vi "ReadWrite.ProcessData.vi"(8 "error in (no error)":errorcluster, 10 "timeout ms":i32=100, 11 "ReadWrite in":refnum<class "ReadWrite.lvclass">) -> (0 "error out":errorcluster, 1 "Timeout?":bool, 2 "Values":dbl[](array[numeric]), 3 "ReadWrite out":refnum<class "ReadWrite.lvclass">, 5 "Detect?":bool[](array[boolean]))   [LabVIEW 2023, in "Plugin Data Access Engine.lvlib" / "ReadWrite.lvclass"]
uses:
  ReadWrite.lvclass
  ReadWrite.lvclass/ReadWrite.ctl
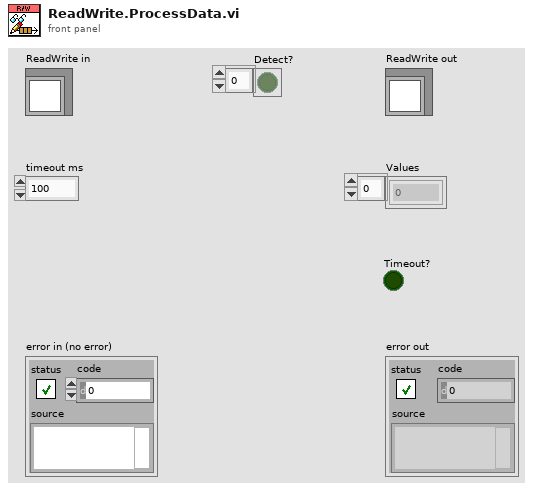
[diagram p1: front panel]
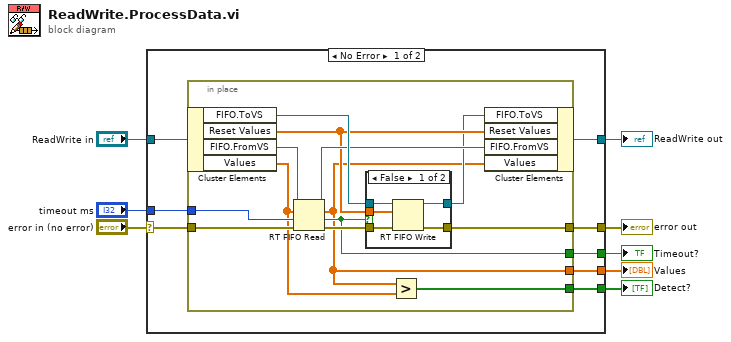
[diagram p0: block diagram]
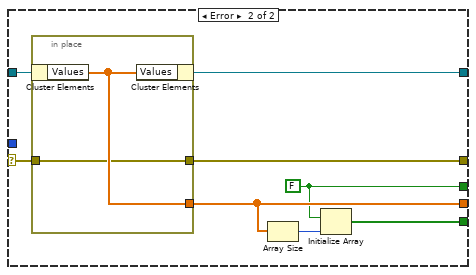
[diagram p3: hidden frame]
diagram:
  n1 = case shown="No Error" "error in (no error)" {
    selector: "error in (no error)" -> [w16 w41]
    tunnel: [w15 w42] -> w7
    tunnel: [w12 w43] -> w5
    tunnel: "ReadWrite in" -> [w13 w44]
    tunnel: [w14 w39] -> w4
    tunnel: "timeout ms" -> [w11 _]
    tunnel: [w10 w37] -> w2
    tunnel: [w9 w38] -> w1
    frame No Error {
      n2 = in-place {
        in-place-border: w16 -> [w28]
        in-place-border: [w22] -> w15
        in-place-border: [w19] -> w14
        in-place-border: w11 -> [w21]
        in-place-border: [w20] -> w10
        in-place-border: [w17] -> w9
        n3 = in-place-cluster #1(w13) -> ("FIFO.ToVS"=w26:refnum<k33>, "Reset Values"=w24:dbl[], "FIFO.FromVS"=w29:refnum<k33>, "Values"=w18:dbl[])
        n4 = RT FIFO Read(0:w29, 1:w18, 2:w21, 3:w28) -> (8:w25:refnum<k33>, 9:w19:dbl[], 10:w20:bool, 11:w27:errorcluster)  [unwired: 1 out]
        n5 = case shown="False" w20 {
          tunnel: w27 -> [w34 w35]
          tunnel: w24 -> [w33 _]
          tunnel: w26 -> [w32 w36]
          tunnel: [w31 w36] -> w23
          tunnel: [w30 w35] -> w22
          frame False {
            n6 = RT FIFO Write(0:w32, 1:w33, 3:w34) -> (8:w31:refnum<k33>, 11:w30:errorcluster)  [unwired: 2 in, 2 out]
          }
          frame True {
          }
        }
        n7 = Greater?(x=w19, y=w18) -> (0:w17:bool[])
        n8 = in-place-cluster #1("FIFO.ToVS"=w23, "Reset Values"=w24, "FIFO.FromVS"=w25, "Values"=w19) -> (w12:refnum<class "ReadWrite.lvclass">)
      }
    }
    frame Error {
      w37 = FALSE ("empty?")
      n9 = in-place {
        in-place-border: [w46] -> w39
        in-place-border: [w45] -> w42
        in-place-border: w41 -> [w45]
        n10 = in-place-cluster #2(w44) -> ("Values"=w46:dbl[])
        n11 = in-place-cluster #2("Values"=w46) -> (w43:refnum<class "ReadWrite.lvclass">)
      }
      n12 = Array Size(array=w39) -> (size(s)=w40:i32)
      n13 = Initialize Array(w37, w40) -> (w38:bool[])
    }
  }
  "error out" <- w7
  "ReadWrite out" <- w5
  "Values" <- w4
  "Timeout?" <- w2
  "Detect?" <- w1
